vi "Data Logging.vi"(8 "error in (no error)":errorcluster, 11 "stop?":bool) -> (0 "error out":errorcluster)   [LabVIEW 2011]
uses:
  <vilib>/Platform/TimedLoop/XDataNode/XDataNode.xnode
  <vilib>/Platform/TimedLoop/XDataNode/nitl_modes.ctl
  <vilib>/Platform/TimedLoop/XDataNode/XDNodeRunTimeDep.lvlib
  <vilib>/Platform/TimedLoop/XDataNode/wakeup.ctl
  <vilib>/Platform/TimedLoop/XDataNode/timing_clust.ctl
  <vilib>/Utility/sysdir.llb/System Directory Type.ctl
panel:
  out "Data Cluster":T1
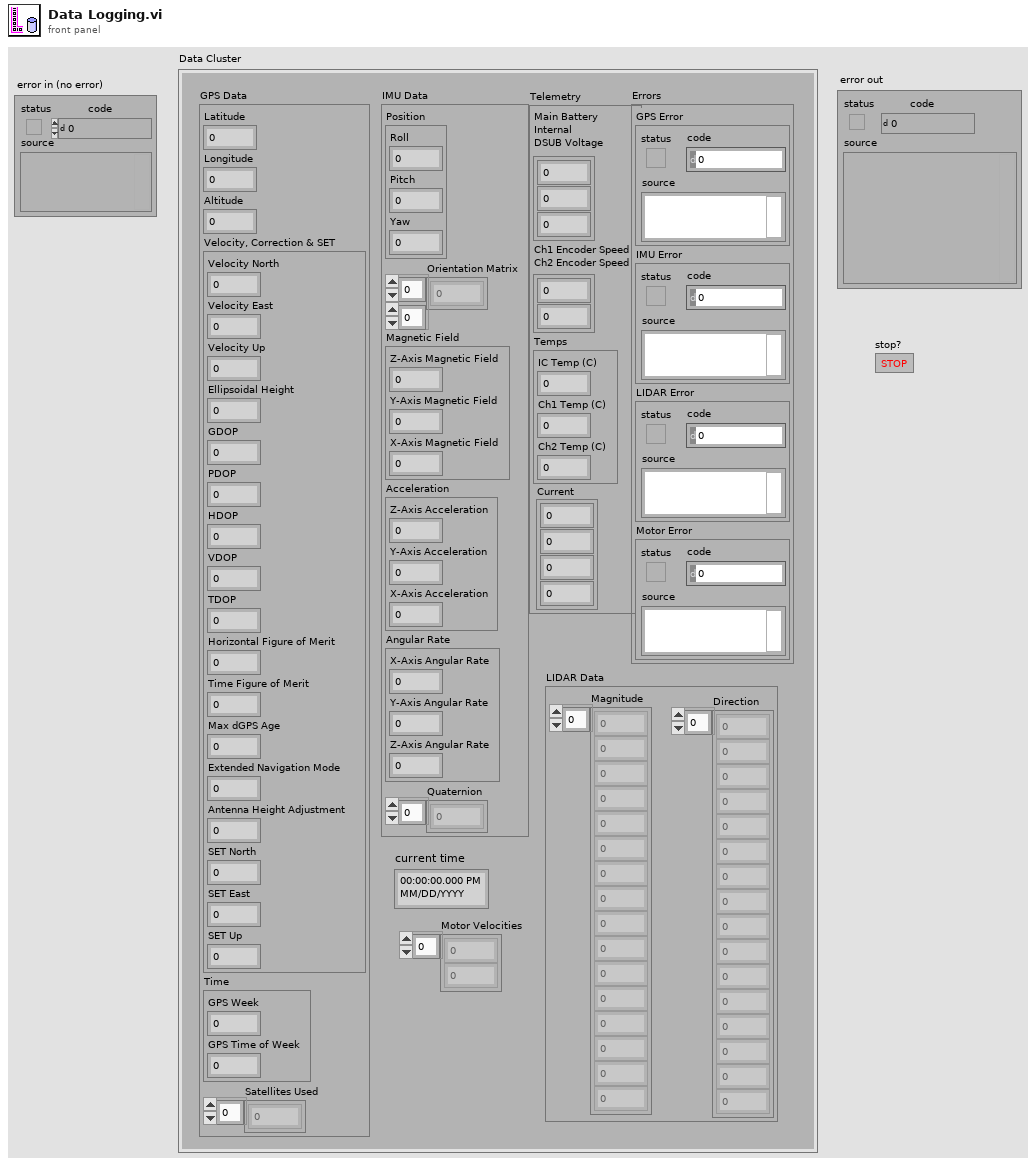
[diagram p1: front panel]
types:
  T1 = cluster{"GPS Data":cluster{"Latitude":dbl, "Longitude":dbl, "Altitude":dbl, "Velocity, Correction & SET":cluster{"Velocity North":dbl, "Velocity East":dbl, "Velocity Up":dbl, "Ellipsoidal Height":dbl, "GDOP":sgl, "PDOP":sgl, "HDOP":sgl, "VDOP":sgl, "TDOP":sgl, "Horizontal Figure of Merit":u8, "Time Figure of Merit":u8, "Max dGPS Age":sgl, "Extended Navigation Mode":u8, "Antenna Height Adjustment ":dbl, "SET North":i32, "SET East":i32, "SET Up":i32}, "Time":cluster{"GPS Week":u16, "GPS Time of Week":sgl}, "Satellites Used":i32[]}, "IMU Data":cluster{"Position":cluster{"Roll":dbl, "Pitch":dbl, "Yaw":dbl}, "Orientation Matrix":dbl[][], "Magnetic Field":cluster{"Z-Axis Magnetic Field":dbl, "Y-Axis Magnetic Field":dbl, "X-Axis Magnetic Field":dbl}, "Acceleration":cluster{"Z-Axis Acceleration":dbl, "Y-Axis Acceleration":dbl, "X-Axis Acceleration":dbl}, "Angular Rate":cluster{"X-Axis Angular Rate":dbl, "Y-Axis Angular Rate":dbl, "Z-Axis Angular Rate":dbl}, "Quaternion":dbl[]}, "Telemetry":cluster{"Main Battery\nInternal\nDSUB Voltage":cluster{sgl, sgl, sgl}, "Ch1 Encoder Speed\nCh2 Encoder Speed":cluster{i32, i32}, "Temps":cluster{"IC Temp (C)":i32, "Ch1 Temp (C)":i32, "Ch2 Temp (C)":i32}, "Current":cluster{dbl, dbl, dbl, dbl}}, "Motor Velocities":dbl[], "Errors":cluster{"GPS Error ":errorcluster, "IMU Error":errorcluster, "LIDAR Error":errorcluster, "Motor Error":errorcluster}, "current time":timestamp, "LIDAR Data":cluster{"Magnitude":dbl[], "Direction":dbl[]}}
  T2 = typedef "System Directory Type.ctl" = i32
  T3 = typedef "XDNodeRunTimeDep.lvlib/timing_clust.ctl" = cluster{"Expected End [f-1]":u64, "Actual End [f-1]":u64, "Finished Late? [f-1]":bool, "Expected End [i-1]":u64, "Actual End [i-1]":u64, "Finished Late? [i-1]":bool, "Expected Start [i]":u64, "Actual Start [i]":u64, "Expected Start [f]":u64, "Actual Start [f]":u64, "Source Name":string, "Structure Name":string, "Period":i64, "Deadline":i64, "Offset":i64, "Start":i64, "Priority":i32, "Timeout":i32, "Mode":T4, "Wakeup Reason":T5, "Error":errorcluster, "Source Type":string, "Secondary Source Type":string, "Global End Time":u64, "Global Start Time":u64, "Frame Duration":u64, "Iteration Duration":u64, "Assigned CPU":i32, "I/O Scan Engine Mode":u32}
  T4 = typedef "XDNodeRunTimeDep.lvlib/nitl_modes.ctl" = enum32{"No Change", "Process missed periods, maintain original phase", "Discard missed periods, maintain original phase", "Process missed periods, ignore original phase", "Discard missed periods, ignore original phase"}
  T5 = typedef "XDNodeRunTimeDep.lvlib/wakeup.ctl" = enum32{"Normal", "Aborted", "Asynchronous wakeup", "Timing source error", "Timed loop error", "Timeout"}
  T6 = cluster{"GPS Error ":errorcluster, "IMU Error":errorcluster, "LIDAR Error":errorcluster, "Motor Error":errorcluster}
  T7 = cluster{"Voltage":cluster{sgl, sgl, sgl}, "Encoder Speed":cluster{i32, i32}, "Temps":cluster{"IC Temp (C)":i32, "Ch1 Temp (C)":i32, "Ch2 Temp (C)":i32}, "Current":cluster{dbl, dbl, dbl, dbl}}
  T8 = cluster{"Latitude":dbl, "Longitude":dbl, "Altitude":dbl, "Velocity, Correction & SET":cluster{"Velocity North":dbl, "Velocity East":dbl, "Velocity Up":dbl, "Ellipsoidal Height":dbl, "GDOP":sgl, "PDOP":sgl, "HDOP":sgl, "VDOP":sgl, "TDOP":sgl, "Horizontal Figure of Merit":u8, "Time Figure of Merit":u8, "Max dGPS Age":sgl, "Extended Navigation Mode":u8, "Antenna Height Adjustment ":dbl, "SET North":i32, "SET East":i32, "SET Up":i32}, "Time":cluster{"GPS Week":u16, "GPS Time of Week":sgl}, "Satellites Used":i32[]}
  T9 = cluster{"Position":cluster{"Roll":dbl, "Pitch":dbl, "Yaw":dbl}, "Orientation Matrix":dbl[][], "Magnetic Field":cluster{"Z-Axis Magnetic Field":dbl, "Y-Axis Magnetic Field":dbl, "X-Axis Magnetic Field":dbl}, "Acceleration":cluster{"Z-Axis Acceleration":dbl, "Y-Axis Acceleration":dbl, "X-Axis Acceleration":dbl}, "Angular Rate":cluster{"X-Axis Angular Rate":dbl, "Y-Axis Angular Rate":dbl, "Z-Axis Angular Rate":dbl}, "Quaternion":dbl[]}
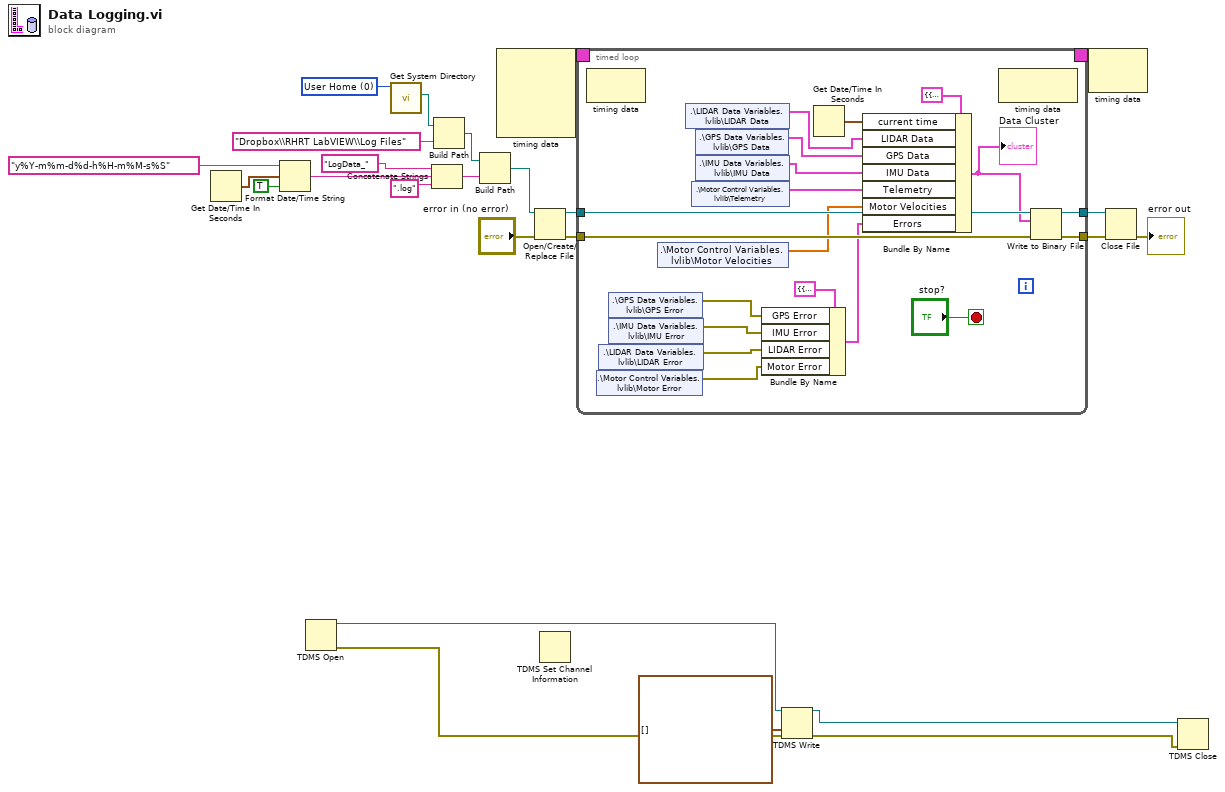
[diagram p0: block diagram]
diagram:
  w16 = T2 0 items=["User Home"=0, "User Desktop"=1, "User Documents"=2, "User Application Data"=3, "User Preferences"=4, "User Temporary"=5, "Public Documents"=6, "Public Application Data"=7, "Public Preferences"=8, "Public Cache"=13, "System Core Libraries"=9, "System Installed Libraries"=10, "Application Files"=11, "Boot Volume Root"=12] ("system directory type")
  n1 = Get Date/Time In Seconds() -> (seconds since 1Jan1904=w22:timestamp)
  n2 = Format Date/Time String(time format string (%c)="y%Y-m%m-d%d-h%H-m%M-s%S", seconds (now)=w22, UTC format=TRUE) -> (date/time string=w20:string)
  n3 = TDMS Open() -> (0:w2:errorcluster, 3:w5:refnum<k34>)  [unwired: 6 in]
  n4 = call <vilib>:"Get System Directory.vi"("system directory type"=w16) -> ("system directory"=w14:path)  [unwired: 10 in]
  n5 = Concatenate Strings("LogData_", w20, ".log") -> (w17:string)
  n6 = Build Path(base path=w14, name or relative path="Dropbox\\RHRT LabVIEW\\Log Files") -> (appended path=w15:path)
  n7 = Build Path(base path=w15, name or relative path=w17) -> (appended path=w9:path)
  n8 = node-c288() -> (w25:T3)  [unwired: 4 in]
  n9 = Open/Create/Replace File(file path (use dialog)=w9, error in="error in (no error)") -> (refnum out=w10:refnum<file>, error out=w11:errorcluster)  [unwired: 4 in, 1 out]
  n10 = TDMS Set Channel Information() -> ()  [unwired: 7 in, 2 out]
  n11 = timed-loop {
    timing: w25 -> [_]
    timing-out: [_] -> w24
    tunnel: w10 -> [w38]
    tunnel: [w36] -> w8
    tunnel: w11 -> [w37]
    tunnel: [w28] -> w6
    stop <- "stop?" stop-if-true
    n12 = node-c288() -> ()  [unwired: 1 in, 1 out]
    n13 = shared-variable ".\\Motor Control Variables.lvlib\\Motor Error"() -> (w44:errorcluster)  [unwired: 1 in, 1 out]
    n14 = shared-variable ".\\LIDAR Data Variables.lvlib\\LIDAR Error"() -> (w43:errorcluster)  [unwired: 1 in, 1 out]
    n15 = shared-variable ".\\GPS Data Variables.lvlib\\GPS Error"() -> (w41:errorcluster)  [unwired: 1 in, 1 out]
    n16 = shared-variable ".\\IMU Data Variables.lvlib\\IMU Error"() -> (w42:errorcluster)  [unwired: 1 in, 1 out]
    n17 = shared-variable ".\\Motor Control Variables.lvlib\\Motor Velocities"() -> (w34:dbl[])  [unwired: 1 in, 1 out]
    n18 = shared-variable ".\\LIDAR Data Variables.lvlib\\LIDAR Data"() -> (w27:cluster{"Magnitude":dbl[], "Direction":dbl[]})  [unwired: 1 in, 1 out]
    n19 = shared-variable ".\\Motor Control Variables.lvlib\\Telemetry"() -> (w32:T7)  [unwired: 1 in, 1 out]
    n20 = shared-variable ".\\GPS Data Variables.lvlib\\GPS Data"() -> (w30:T8)  [unwired: 1 in, 1 out]
    n21 = shared-variable ".\\IMU Data Variables.lvlib\\IMU Data"() -> (w31:T9)  [unwired: 1 in, 1 out]
    n22 = Bundle By Name(cluster=T6 {"GPS Error "={"status"=FALSE, "code"=0, "source"=""}, "IMU Error"={"status"=FALSE, "code"=0, "source"=""}, "LIDAR Error"={"status"=FALSE, "code"=0, "source"=""}, "Motor Error"={"status"=FALSE, "code"=0, "source"=""}} ("Errors"), "GPS Error"=w41, "IMU Error"=w42, "LIDAR Error"=w43, "Motor Error"=w44) -> (w35:T6)
    n23 = Get Date/Time In Seconds() -> (seconds since 1Jan1904=w26:timestamp)
    n24 = Bundle By Name(cluster=T1 {"GPS Data"={"Latitude"=0.0, "Longitude"=0.0, "Altitude"=0.0, "Velocity, Correction & SET"={"Velocity North"=0.0, "Velocity East"=0.0, "Velocity Up"=0.0, "Ellipsoidal Height"=0.0, "GDOP"=0.0, "PDOP"=0.0, "HDOP"=0.0, "VDOP"=0.0, "TDOP"=0.0, "Horizontal Figure of Merit"=0, "Time Figure of Merit"=0, "Max dGPS Age"=0.0, "Extended Navigation Mode"=0, "Antenna Height Adjustment "=0.0, "SET North"=0, "SET East"=0, "SET Up"=0}, "Time"={"GPS Week"=0, "GPS Time of Week"=0.0}, "Satellites Used"=[]}, "IMU Data"={"Position"={"Roll"=0.0, "Pitch"=0.0, "Yaw"=0.0}, "Orientation Matrix"=[], "Magnetic Field"={"Z-Axis Magnetic Field"=0.0, "Y-Axis Magnetic Field"=0.0, "X-Axis Magnetic Field"=0.0}, "Acceleration"={"Z-Axis Acceleration"=0.0, "Y-Axis Acceleration"=0.0, "X-Axis Acceleration"=0.0}, "Angular Rate"={"X-Axis Angular Rate"=0.0, "Y-Axis Angular Rate"=0.0, "Z-Axis Angular Rate"=0.0}, "Quaternion"=[]}, "Telemetry"={"Main Battery\nInternal\nDSUB Voltage"={0.0, 0.0, 0.0}, "Ch1 Encoder Speed\nCh2 Encoder Speed"={0, 0}, "Temps"={"IC Temp (C)"=0, "Ch1 Temp (C)"=0, "Ch2 Temp (C)"=0}, "Current"={0.0, 0.0, 0.0, 0.0}}, "Motor Velocities"=[], "Errors"={"GPS Error "={"status"=FALSE, "code"=0, "source"=""}, "IMU Error"={"status"=FALSE, "code"=0, "source"=""}, "LIDAR Error"={"status"=FALSE, "code"=0, "source"=""}, "Motor Error"={"status"=FALSE, "code"=0, "source"=""}}, "current time"=timestamp(0 s since 1904-01-01), "LIDAR Data"={"Magnitude"=[], "Direction"=[]}} ("Data Cluster"), "current time"=w26, "LIDAR Data"=w27, "GPS Data"=w30, "IMU Data"=w31, "Telemetry"=w32, "Motor Velocities"=w34, "Errors"=w35) -> (w29:T1)
    "Data Cluster" <- w29
    n25 = node-c288() -> ()  [unwired: 1 in, 1 out]
    n26 = Write to Binary File(file (use dialog)=w38, data=w29, error in=w37) -> (refnum out=w28:refnum<file>, error out=w36:errorcluster)  [unwired: 3 in, 1 out]
  }
  n27 = TDMS Write(0:w5, 9:waveform(dbl)[] [] ("data"), 11:w2) -> (4:w4:refnum<k34>, 15:w3:errorcluster)  [unwired: 3 in, 2 out]
  n28 = node-c288(w24) -> ()  [unwired: 1 out]
  n29 = Close File(refnum=w6, error in=w8) -> (error out=→"error out":errorcluster)  [unwired: 1 out]
  n30 = TDMS Close(8:w3, 11:w4) -> ()  [unwired: 2 out]
